vi "UpItem__slk_tc.vi"(0 "tree control in":refnum<class "TreeControl.lvclass">, 5 "indent tag (current tag)":string, 11 "error in (no error)":errorcluster) -> (4 "tree control out":refnum<class "TreeControl.lvclass">, 15 "error out":errorcluster)   [LabVIEW 2020, in "TreeControl.lvclass"]
doc: "Moves the input tag item upper."
uses:
  Library/TreeControl.lvclass
  Library/TreeControl.lvclass/TreeControl.ctl
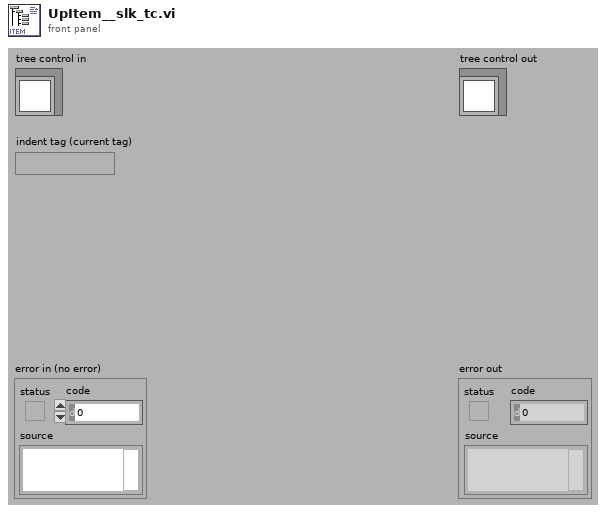
[diagram p1: front panel]
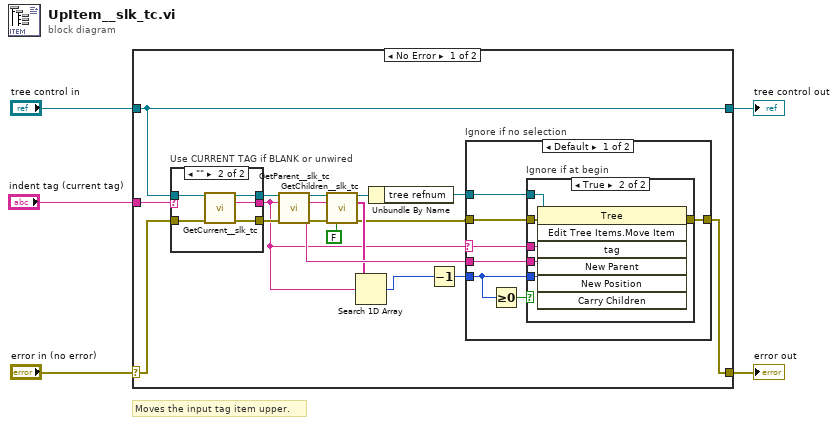
[diagram p0: block diagram]
diagram:
  # "Moves the input tag item upper."
  n1 = case shown="No Error" "error in (no error)" {
    selector: "error in (no error)" -> [w10 w47]
    tunnel: [w9 w47] -> w4
    tunnel: [w22 w46] -> w2
    tunnel: "tree control in" -> [w22 w46]
    tunnel: "indent tag (current tag)" -> [w8 _]
    frame No Error {
      n2 = case "Use CURRENT TAG if BLANK or unwired" shown="\"\"" w8 {
        selector: w8 -> [w40 _]
        tunnel: [w40 w45] -> w13
        tunnel: w22 -> [w38 w44]
        tunnel: w10 -> [w39 w43]
        tunnel: [w39 w42] -> w19
        tunnel: [w38 w41] -> w20
        frame Default {
        }
        frame "" {
          n3 = call "GetCurrent__slk_tc.vi"("tree control in"=w44, "error in (no error)"=w43) -> ("tree control out"=w41:refnum<class "TreeControl.lvclass">, "current tag"=w45:string, "error out"=w42:errorcluster)  [unwired: 1 in, 10 out]
        }
      }
      n4 = call "GetParent__slk_tc.vi"("tree control in"=w20, "child tag (\"\")"=w13, "error in (no error)"=w19) -> ("tree control out"=w18:refnum<class "TreeControl.lvclass">, "parent tag"=w16:string, "error out"=w17:errorcluster)  [unwired: 10 out]
      n5 = call "GetChildren__slk_tc.vi"("tree control in"=w18, "parent tag (\"\")"=w16, "error in (no error)"=w17, "use current (T)"=FALSE) -> ("tree control out"=w14:refnum<class "TreeControl.lvclass">, "children tags"=w15:string[], "error out"=w11:errorcluster)  [unwired: 9 out]
      n6 = Search 1D Array(1D array=w15, element=w13) -> (index of element=w12:i32)  [unwired: 1 out]
      n7 = Unbundle By Name(w14) -> ("tree refnum"=w21:refnum<vi>)
      n8 = Decrement(x=w12) -> (x-1=w6:i32)
      n9 = case "Ignore if no selection" shown="Default" w13 {
        selector: w13 -> [w28 _]
        tunnel: w21 -> [w27 _]
        tunnel: w11 -> [w29 w37]
        tunnel: [w26 w37] -> w9
        tunnel: w16 -> [w25 _]
        tunnel: w6 -> [w24 _]
        frame Default {
          n10 = Greater Or Equal To 0?(x=w24) -> (x >= 0?=w23:bool)
          n11 = case "Ignore if at begin" shown="True" w23 {
            tunnel: w29 -> [w30 w36]
            tunnel: w28 -> [_ w35]
            tunnel: w27 -> [_ w34]
            tunnel: [w30 w33] -> w26
            tunnel: w25 -> [_ w32]
            tunnel: w24 -> [_ w31]
            frame False {
            }
            frame True {
              n12 = invoke class="Tree" method="Edit Tree Items.Move Item"(reference=w34, error in=w36, "tag"=w35, "New Parent"=w32, "New Position"=w31) -> (error out=w33:errorcluster)  [unwired: 2 in, 6 out]
            }
          }
        }
        frame "" {
        }
      }
    }
    frame Error {
    }
  }
  "error out" <- w4
  "tree control out" <- w2
